vi "Serial.vi"(2 "VISA resource name":refnum<visa-resource-name>) -> (5 "VISA resource name out":refnum<visa-resource-name>, 6 "Serial Configuration Out":T1={"Baud Rate"=9600, "Parity"=0, "Data Bits"=8, "Stop Bits"=10, "Flow Control"=0} {"Flow Control" items=["None", "XON/XOFF", "RTS/CTS", "XON/XOFF & RTS/CTS", "DTR/DSR", "XON/XOFF & DTR/DSR"]; "Stop Bits" items=["1.0"=10, "1.5"=15, "2.0"=20]; "Data Bits" items=["7"=7, "8"=8]; "Parity" items=["None", "Odd", "Even", "Mark", "Space"]; "Baud Rate" items=["300"=300, "600"=600, "1200"=1200, "2400"=2400, "4800"=4800, "9600"=9600, "19200"=19200]}, 7 "semaphore":T2, 8 "Serial error out":errorcluster)   [LabVIEW 2018, in "com.Instrument.lvlib"]
uses:
  com.Instrument.lvlib
panel:
  in  "Serial Configuration":T1={"Baud Rate"=9600, "Parity"=0, "Data Bits"=8, "Stop Bits"=10, "Flow Control"=0} {"Flow Control" items=["None", "XON/XOFF", "RTS/CTS", "XON/XOFF & RTS/CTS", "DTR/DSR", "XON/XOFF & DTR/DSR"]; "Stop Bits" items=["1.0"=10, "1.5"=15, "2.0"=20]; "Data Bits" items=["7"=7, "8"=8]; "Parity" items=["None", "Odd", "Even", "Mark", "Space"]; "Baud Rate" items=["300"=300, "600"=600, "1200"=1200, "2400"=2400, "4800"=4800, "9600"=9600, "19200"=19200]}
  in  "Serial error in (no error)":errorcluster
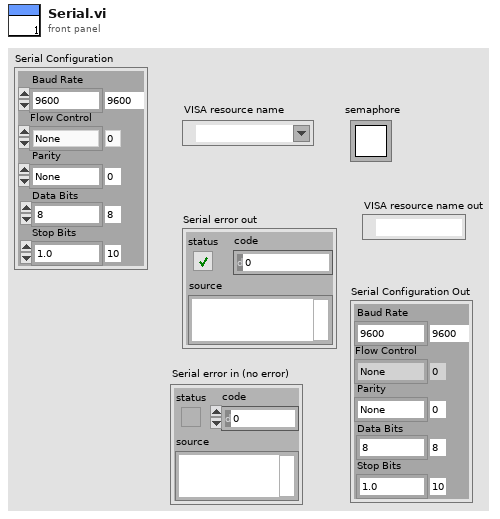
[diagram p1: front panel]
types:
  T1 = cluster{"Baud Rate":u32, "Parity":u16, "Data Bits":u16, "Stop Bits":u16, "Flow Control":u16}
  T2 = typedef "Semaphore RefNum" = refnum<k1>
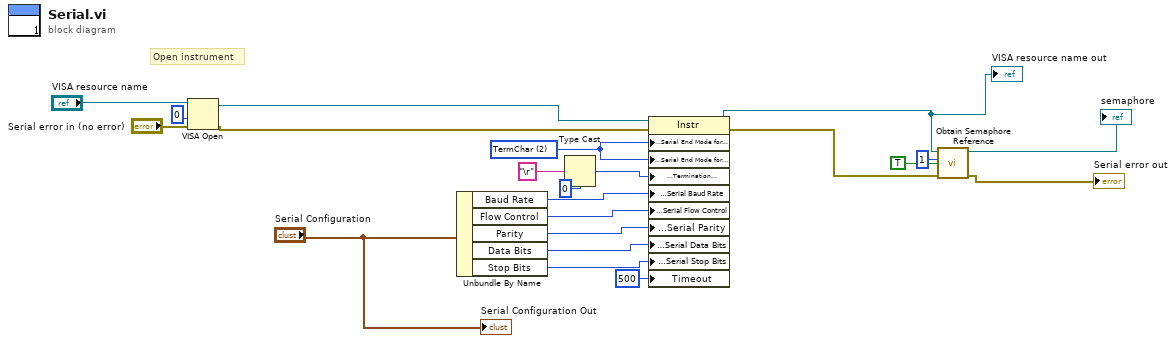
[diagram p0: block diagram]
diagram:
  w8 = u16 2 items=["None", "LastBit", "TermChar"] ("Serial Settings:Serial End Mode for Reads")
  # "Open instrument"
  n1 = VISA Open(access mode=u32 0, error in (no error)="Serial error in (no error)", VISA resource name="VISA resource name") -> (VISA resource name=w7:refnum<visa-resource-name>, error out=w6:errorcluster)  [unwired: 2 in]
  n2 = Unbundle By Name("Serial Configuration") -> ("Baud Rate"=w13:u32, "Flow Control"=w10:u16, "Parity"=w11:u16, "Data Bits"=w12:u16, "Stop Bits"=w9:u16)
  n3 = Type Cast(type=u8 0, x="\r") -> (*(type *) &x=w4:u8)
  n4 = property class="Instr"(reference=w7, error in=w6, "Serial Settings:Serial End Mode for Reads"=w8, "Serial Settings:Serial End Mode for Writes"=w8, "Message Based Settings:Termination Character"=w4, "Serial Settings:Serial Baud Rate"=w13, "Serial Settings:Serial Flow Control"=w10, "Serial Settings:Serial Parity"=w11, "Serial Settings:Serial Data Bits"=w12, "Serial Settings:Serial Stop Bits"=w9, "Timeout"=u32 500 ("General Settings:Timeout Value")) -> (reference out=w2:refnum<visa-resource-name>, error out=w3:errorcluster)
  "VISA resource name out" <- w2
  n5 = call <vilib>:"Obtain Semaphore Reference.vi"("error in (no error)"=w3, "create if not found (T)"=TRUE, "size (1)"=1, "name (unnamed)"=w2) -> ("error out"=→"Serial error out":errorcluster, "semaphore"=→"semaphore":T2)  [unwired: 1 in, 1 out]
  "Serial Configuration Out" <- "Serial Configuration"
